vi "Read NET_StreamContent.vi"(8 "error in (no error)":errorcluster, 11 "HttpContent_Stream in":refnum<class "HttpContent_Stream.lvclass">) -> (0 "error out":errorcluster, 2 "NET_StreamContent":refnum<k24>, 3 "HttpContent_Stream out":refnum<class "HttpContent_Stream.lvclass">)   [LabVIEW 2018, in "HttpClient_NET.lvlib" / "HttpContent_Stream.lvclass"]
doc: "<b> </b> <b> </b>\nHttpClient_NET\nJustin Young - Viviota\nCopyright (c) 2021\nLicense: BSD"
uses:
  HttpContent_Stream.lvclass
  C:/Viviota/Projects/R&D/__OpenSource/VIV_HTTP_REST_NET/HttpContent/HttpContent.lvclass
  System.Net.Http
  HttpContent/HttpContent.lvclass/HttpContent.ctl
  HttpContent/HttpContent.lvclass
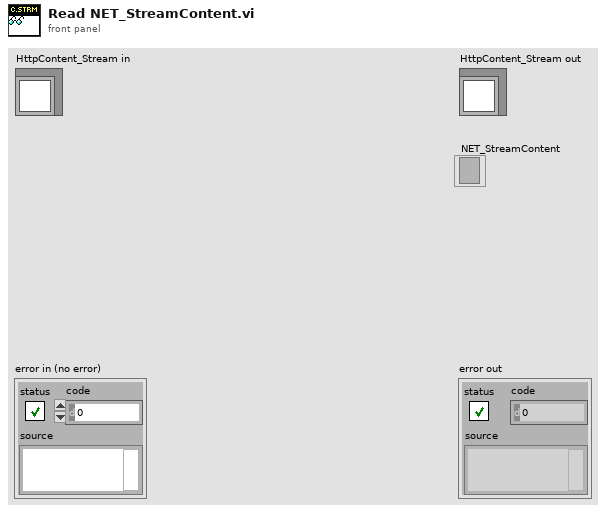
[diagram p1: front panel]
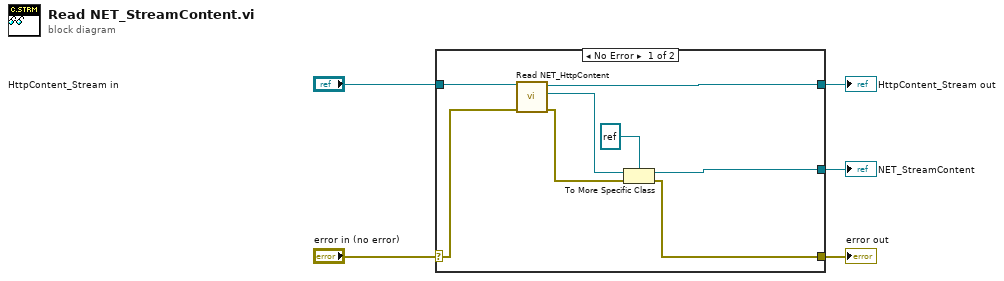
[diagram p0: block diagram]
diagram:
  n1 = case shown="No Error" "error in (no error)" {
    selector: "error in (no error)" -> [w7 w14]
    tunnel: [w6 w14] -> w4
    tunnel: [w10 w15] -> w2
    tunnel: "HttpContent_Stream in" -> [w11 w15]
    tunnel: [w8 _] -> w1
    frame No Error {
      n2 = call "Read NET_HttpContent.vi"("error in (no error)"=w7, "HttpContent in"=w11) -> ("error out"=w13:errorcluster, "NET_HttpContent"=w12:refnum<k24>, "HttpContent out"=w10:refnum<class "HttpContent_Stream.lvclass">)  [unwired: 7 in]
      n3 = To More Specific Class(target class=refnum<k24> refnum ("NET_StreamContent"), reference=w12, error in=w13) -> (specific class reference=w8:refnum<k24>, error out=w6:errorcluster)
    }
    frame Error {
    }
  }
  "error out" <- w4
  "HttpContent_Stream out" <- w2
  "NET_StreamContent" <- w1
